vi "The library at a glance.vi"   [LabVIEW 2018, in "status_text_indicator.lvlib"]
uses:
  status_text_indicator.lvlib
  PTRL/String_Control/string_control.lvlib
panel:
  # "status_text_indicator library at a glance"
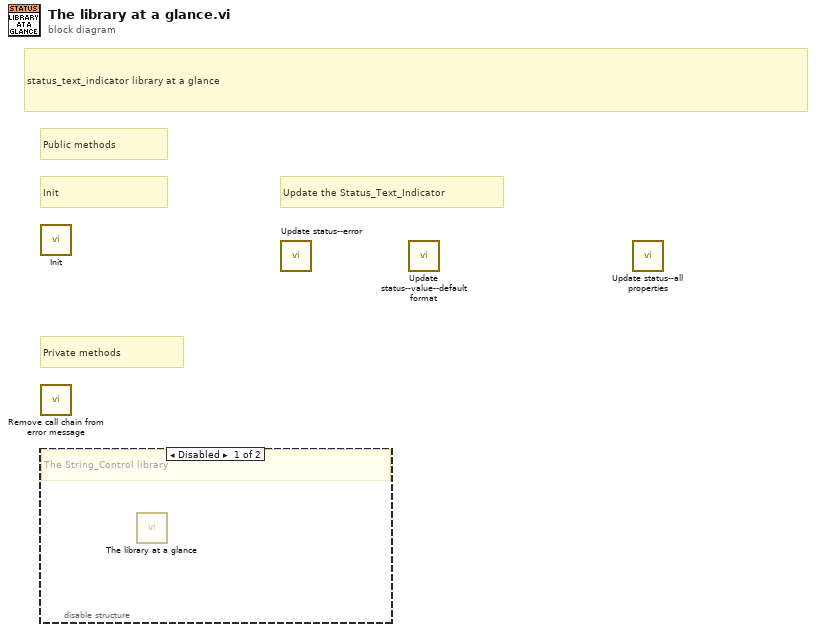
[diagram p0: block diagram]
diagram:
  # "Public methods"
  # "Private methods"
  # "Update the Status_Text_Indicator"
  # "Init"
  # "status_text_indicator library at a glance"
  n1 = call "Init.vi"() -> ()  [unwired: 11 in, 1 out]
  n2 = call "Remove call chain from error message.vi"() -> ()  [unwired: 1 in, 1 out]
  n3 = disable-structure shown="Disabled" {
    frame Disabled {
      # "The String_Control library"
      n4 = call "The library at a glance.vi"() -> ()  [unwired: 12 in]
    }
    frame Enabled {
    }
  }
  n5 = call "Update status--error.vi"() -> ()  [unwired: 11 in, 1 out]
  n6 = call "Update status--value--default format.vi"() -> ()  [unwired: 11 in, 1 out]
  n7 = call "Update status--all properties.vi"() -> ()  [unwired: 11 in, 1 out]
